vi "Blocking Performance Test Application Globals.vi"() -> ()   [LabVIEW 2013]
panel:
  in  "Test Paramaters File Name":string="BlockingTests.ini"
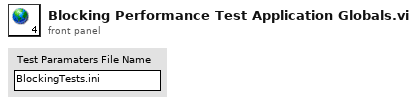
[diagram p1: front panel]
diagram:
